vi "to_json.vi"(8 "error in":errorcluster, 11 "all in":refnum<class "all.lvclass">) -> (0 "error out":errorcluster, 2 "json":string, 3 "all out":refnum<class "all.lvclass">, 4 "Not Default":bool)   [LabVIEW 2020, in "nominal types.lvlib" / "channelFilter.lvlib" / "all.lvclass"]
uses:
  all.lvclass
  6d611ec1-bcaa-4bca-b46d-5e409a1cfc52.vi
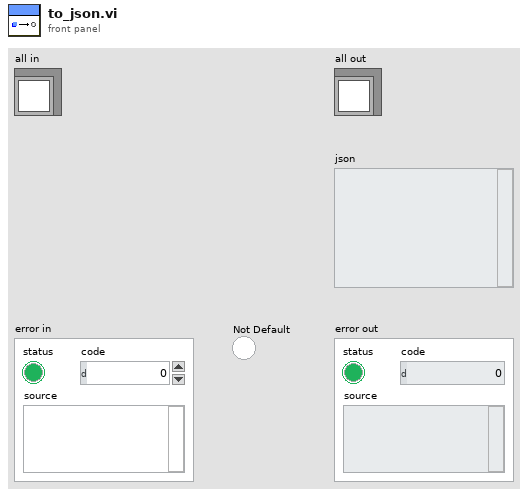
[diagram p1: front panel]
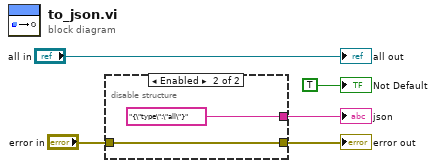
[diagram p0: block diagram]
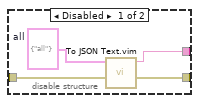
[diagram p2: hidden frame]
diagram:
  n1 = disable-structure shown="Enabled" {
    disable-tunnel: [w9 "{\"type\":\"all\"}" ("json")] -> w4
    disable-tunnel: [w8 w10] -> w3
    disable-tunnel: "error in" -> [w7 w10]
    frame Disabled {
      w6 = cluster{"type":string} {"type"="all"}  # all
      n2 = call "To JSON Text.vim"("error in (no error)"=w7, "Anything"=w6) -> ("error out"=w8:errorcluster, "<JSON>"=w9:string)  [unwired: 8 in]
    }
    frame Enabled {
    }
  }
  "error out" <- w3
  "json" <- w4
  "all out" <- "all in"
  "Not Default" <- TRUE ("Not Default")
